vi "Pcre2SetOptimize8.vi"(8 "error in":errorcluster, 10 "OptimizeDirective":u32, 11 "pCompileContext":u64 format="%.0x") -> (0 "error out":errorcluster, 3 "pCompileContext":u64 format="%.0x")   [LabVIEW 2021, in "libpcre2-8.lvlib"]
uses:
  libpcre2-8.lvlib
  libpcre2-8-x32.dll
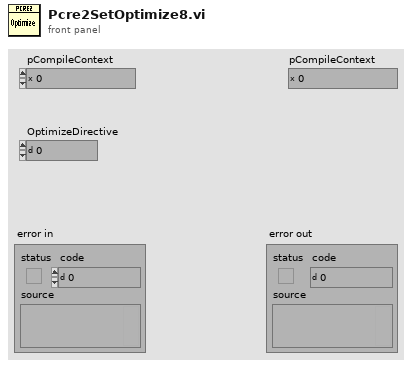
[diagram p1: front panel]
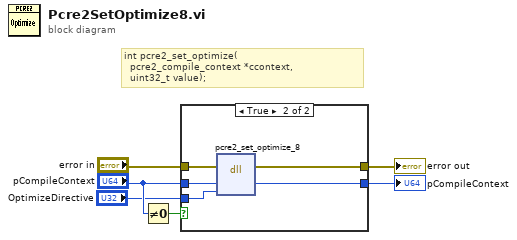
[diagram p0: block diagram]
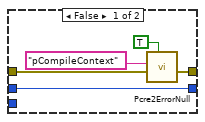
[diagram p2: hidden frame]
diagram:
  # "int pcre2_set_optimize(\n  pcre2_compile_context *ccontext,\n  uint32_t value);"
  n1 = Not Equal To 0?(x="pCompileContext") -> (x != 0?=w1:bool)
  n2 = case shown="True" w1 {
    tunnel: "error in" -> [w10 w16]
    tunnel: [w11 w15] -> w5
    tunnel: "OptimizeDirective" -> [_ w14]
    tunnel: "pCompileContext" -> [w8 w13]
    tunnel: [w8 w12] -> w4
    frame False {
      n3 = call "Pcre2ErrorNull.vi"("IsPointer? (F)"=TRUE, "error in"=w10, "What"="pCompileContext") -> ("error out"=w11:errorcluster)  [unwired: 8 in]
    }
    frame True {
      n4 = dll-call lib="libpcre2-8-x*.dll" fn="pcre2_set_optimize_8"(error in=w16, "ccontext"=w13, "directive"=w14) -> (error out=w15:errorcluster, "ccontext"=w12:u64)  [unwired: 4 in, 1 out]
    }
  }
  "error out" <- w5
  "pCompileContext" <- w4
